vi "wait on clock.vi"(8 "error in":errorcluster, 10 "dt":u32=1, 11 "timing source in":refnum<class "absolute usec timing source.lvclass">) -> (0 "error out":errorcluster, 2 "ticks since last call":u32, 3 "timing source out":refnum<class "absolute usec timing source.lvclass">)   [LabVIEW 2013, in "absolute usec timing source.lvclass"]
doc: "This core timing function is used inside of a loop to wait for a clock signal, or dt ticks of a clock signal."
uses:
  absolute usec timing source.lvclass
  absolute usec timing source.lvclass/absolute usec timing source.ctl
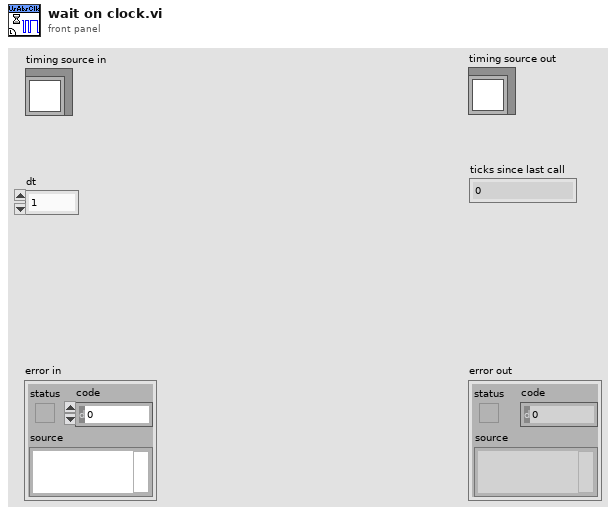
[diagram p1: front panel]
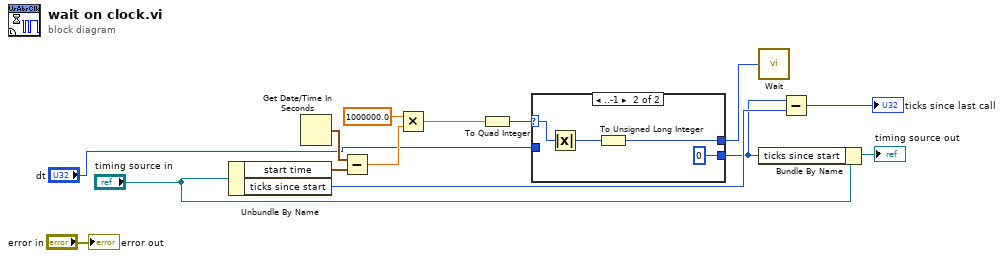
[diagram p0: block diagram]
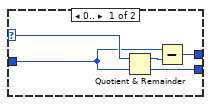
[diagram p2: hidden frame]
diagram:
  n1 = Unbundle By Name("timing source in") -> ("start time"=w13:timestamp, "ticks since start"=w6:i64)
  n2 = Get Date/Time In Seconds() -> (seconds since 1Jan1904=w12:timestamp)
  n3 = Subtract(x=w12, y=w13) -> (x-y=w11:dbl)
  n4 = Multiply(x=1000000.0, y=w11) -> (x*y=w9:dbl)
  n5 = To Quad Integer(1:w9) -> (0:w8:i64)
  n6 = case shown="..-1" w8 {
    selector: w8 -> [w19 w23]
    tunnel: "dt" -> [w17 _]
    tunnel: [w16 w21] -> w7
    tunnel: [w15 i64 0] -> w5
    frame 0.. {
      n7 = Quotient & Remainder(x=w19, y=w17) -> (x-y*floor(x/y)=w18:i64, floor(x/y)=w15:i64)
      n8 = Subtract(x=w17, y=w18) -> (x-y=w16:u32)
    }
    frame ..-1 {
      n9 = Absolute Value(x=w23) -> (abs(x)=w22:i64)
      n10 = To Unsigned Long Integer(number=w22) -> (unsigned 32bit integer=w21:u32)
    }
  }
  n11 = call "Wait"("Count(uSec)"=w7) -> ()  [unwired: 1 out]
  n12 = Bundle By Name(cluster="timing source in", "ticks since start"=w5) -> (→"timing source out":refnum<class "absolute usec timing source.lvclass">)
  n13 = Subtract(x=w5, y=w6) -> (x-y=→"ticks since last call":u32)
  "error out" <- "error in"
